vi "RH - PSTC MHCB2 SOFTWARE 2.0.vi"() -> ()   [LabVIEW 2021]
uses:
  Controls/Queue steps Main applic.ctl
  Controls/ApplicSettings.ctl
  <vilib>/Utility/miscctls.llb/LVRectTypeDef.ctl
  Error notification/Controls/Error notification - Settings.ctl
  Error notification/Controls/Error notification - shown buttons.ctl
  Controls/Initialized boards information.ctl
  MDI handling/Controls/MDI FG registered windows states.ctl
  MDI handling/Controls/MDI Arrange child in parent states.ctl
  MDI handling/MDI global.vi
  Controls/RH PSTC MHCB2 CONSOLE global.vi
  <vilib>/Utility/miscctls.llb/LVPointTypeDef.ctl
panel:
  out "Session loaded":path
  in  "Do not use":bool
  out "close":bool
  out "Opened child ref.":refnum<vi>
  out "Session to load":path
  in  "Debugging info":bool
  out "Child to open":path
  in  "Settings":T1
  in  "Queue steps":T3=enum."idle"
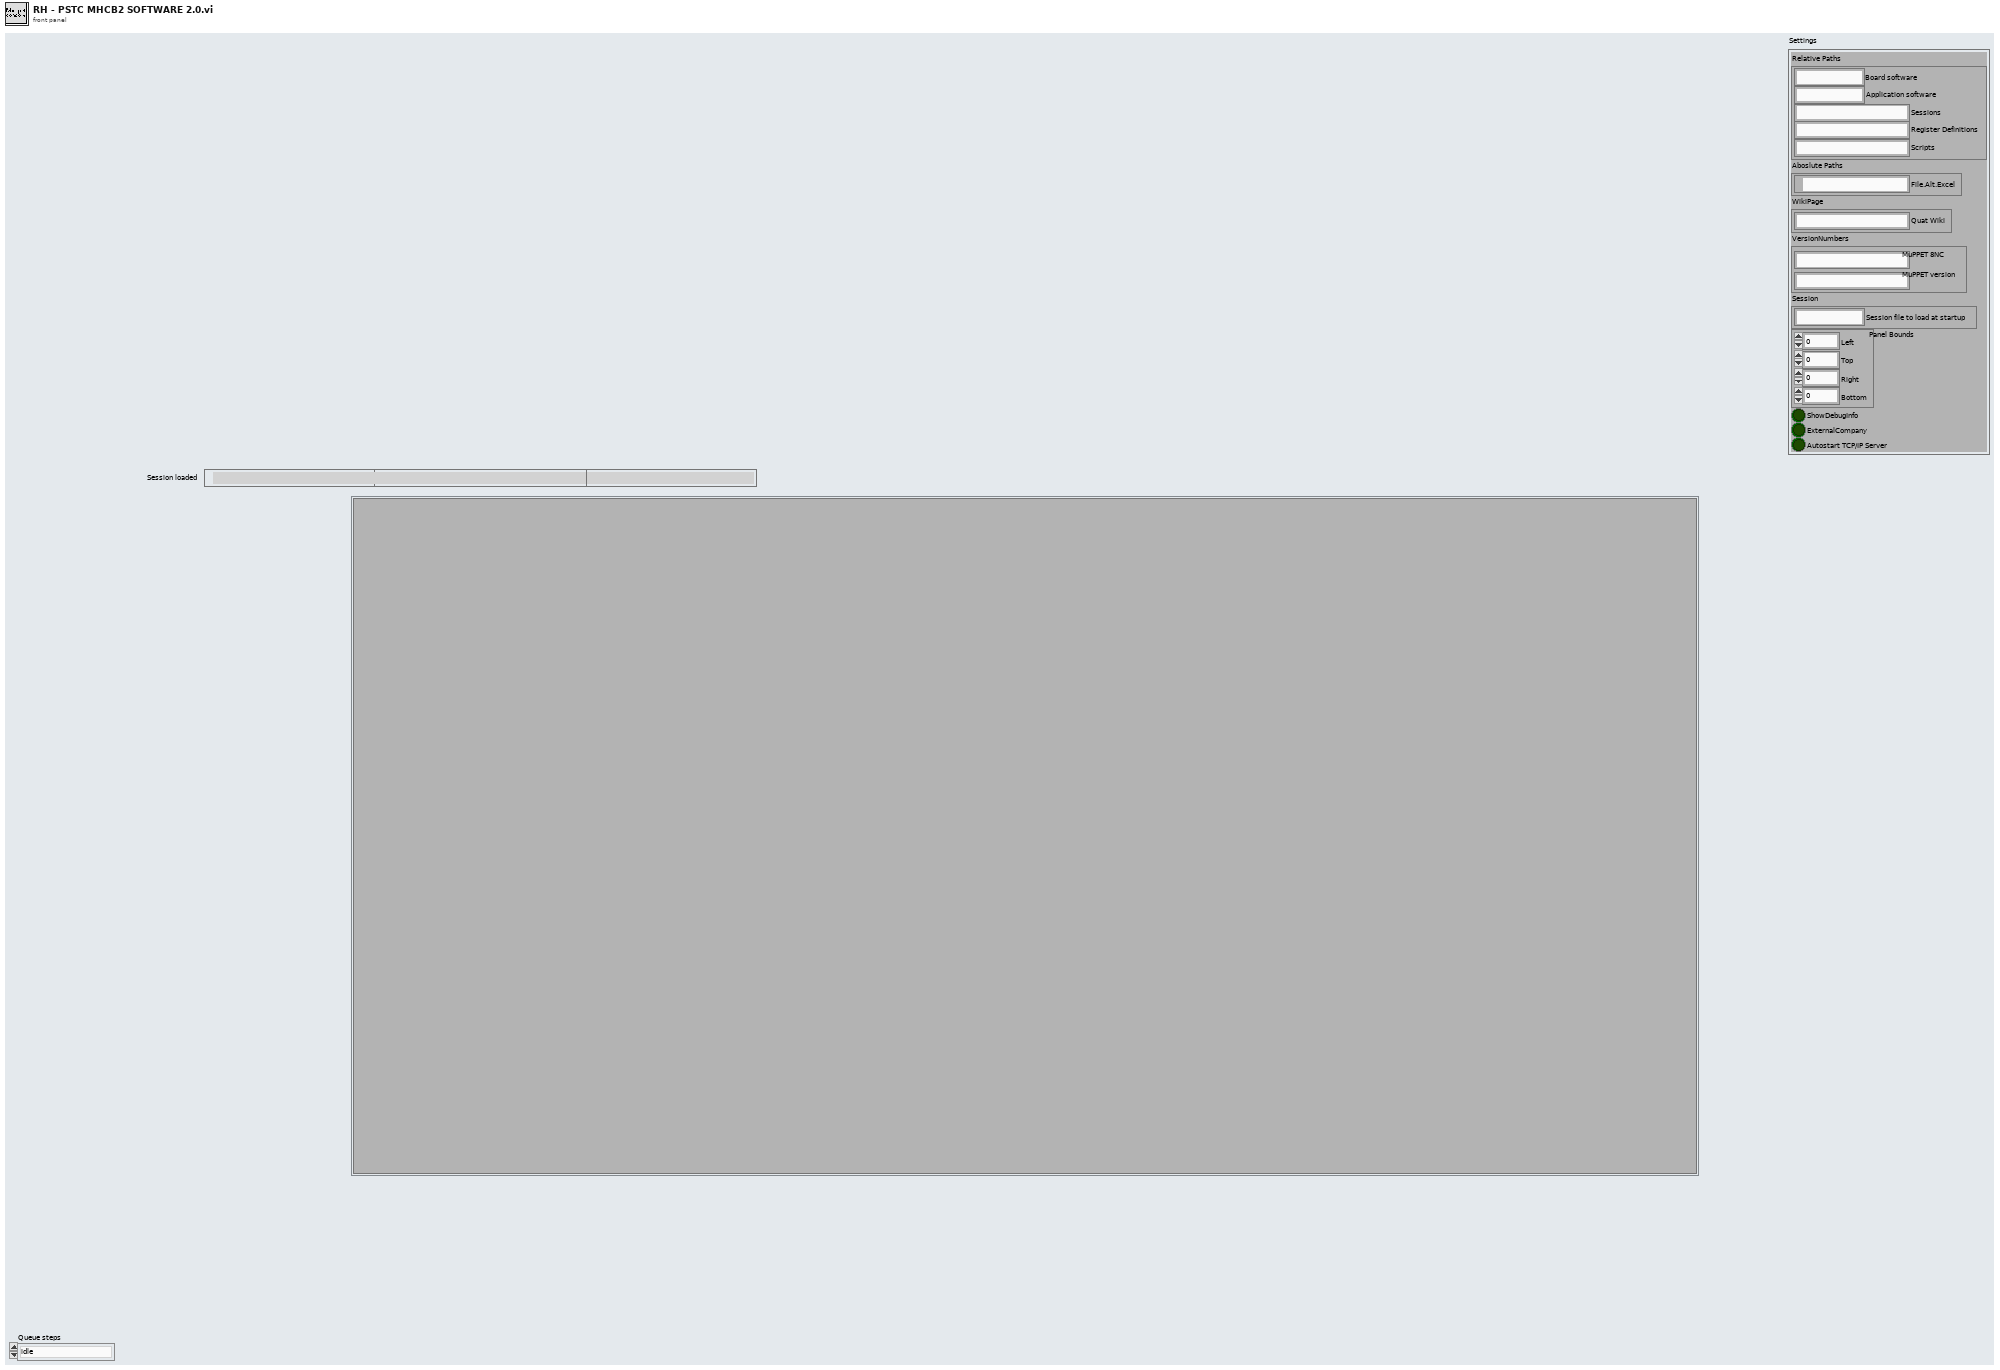
[diagram p1: front panel]
types:
  T1 = typedef "ApplicSettings.ctl" = cluster{"Relative Paths":cluster{"Board software":string, "Application software":string, "Sessions":string, "Register Definitions":string, "Scripts":string}, "Aboslute Paths":cluster{"File.Alt.Excel":path}, "WikiPage":cluster{"Quat Wiki":string}, "VersionNumbers":cluster{"MuPPET 8NC":string, "MuPPET version":string}, "Session":cluster{"Session file to load at startup":string}, "Panel Bounds":T2, "ShowDebugInfo":bool, "ExternalCompany":bool, "Autostart TCP/IP Server":bool}
  T2 = typedef "LVRectTypeDef.ctl" = cluster{"Left":i16, "Top":i16, "Right":i16, "Bottom":i16}
  T3 = typedef "Queue steps Main applic.ctl" = enum16{"init", "idle", "error", "exit", "About", "-----------------", "Startup: Find available software", "Startup: Create pulldown menu", "Startup: Run board SW startup VIs", "File IO: Load applic settings", "File IO: Save applic settings", "MDI: init", "MDI: open child", "MDI: close", "Session: close", "Session: load", "Session: save", "Session: save as", "Hardware: Close", "Script", "TCP IP script server", "Import Excel table layout", "Test: insert error"}
  T4 = enum32{"invalid app kind", "Development System", "Run Time System", "Student Edition", "Embedded LabVIEW", "Evaluation", "Custom"}
  T5 = typedef "Error notification - Settings.ctl" = cluster{"Window Lay-out":cluster{"Title":string, "Show modal":bool, "Default buttons":T6}, "Logging":cluster{"Enable":bool, "Filepath":path, "Max # of lines in file":i32}, "Error definition file":cluster{"Filepath":path}}
  T6 = typedef "Error notification - shown buttons.ctl" = cluster{"Ignore":bool, "Retry":bool, "Abort":bool, "Abort application":bool}
  T7 = typedef "LVPointTypeDef.ctl" = cluster{"Horizontal":i16, "Vertical":i16}
  T8 = typedef "Initialized boards information.ctl" = cluster{"BoardName":string, "Simulation":bool}
  T9 = typedef "MDI FG registered windows states.ctl" = enum16{"init", "add", "replace", "remove", "read"}
  T10 = typedef "MDI Arrange child in parent states.ctl" = enum16{"SW: TopLeft", "SW: Position Coordinated", "SW: Position Incremental", "SW: Center", "SW: Resize", "SW: Resize animated", "AW: Tile", "MW: Arrange Iconic"}
  T11 = cluster{"PositionChildOptions":T10, "X offset":i32, "Y offset":i32}
  T12 = typedef "Error notification - respone.ctl" = enum16{"NOP", "Ignore", "Retry", "Abort", "Abort Applic"}
  T13 = cluster{"IndentLvl":i32, "Type":enum16{"Submenu", "Item", "Separator"}, "Name":string, "Tag":path}[]
  T14 = typedef "MDI child window props.ctl" = cluster{"Owner hWnd":u32, "hWnd":u32, "VI Refnum":refnum<vi>, "WindowTitle":string, "File":string, "Target":string, "RelativeVIPath":string, "PaneState":enum16{"Norm", "Minimized", "Maximized"}}
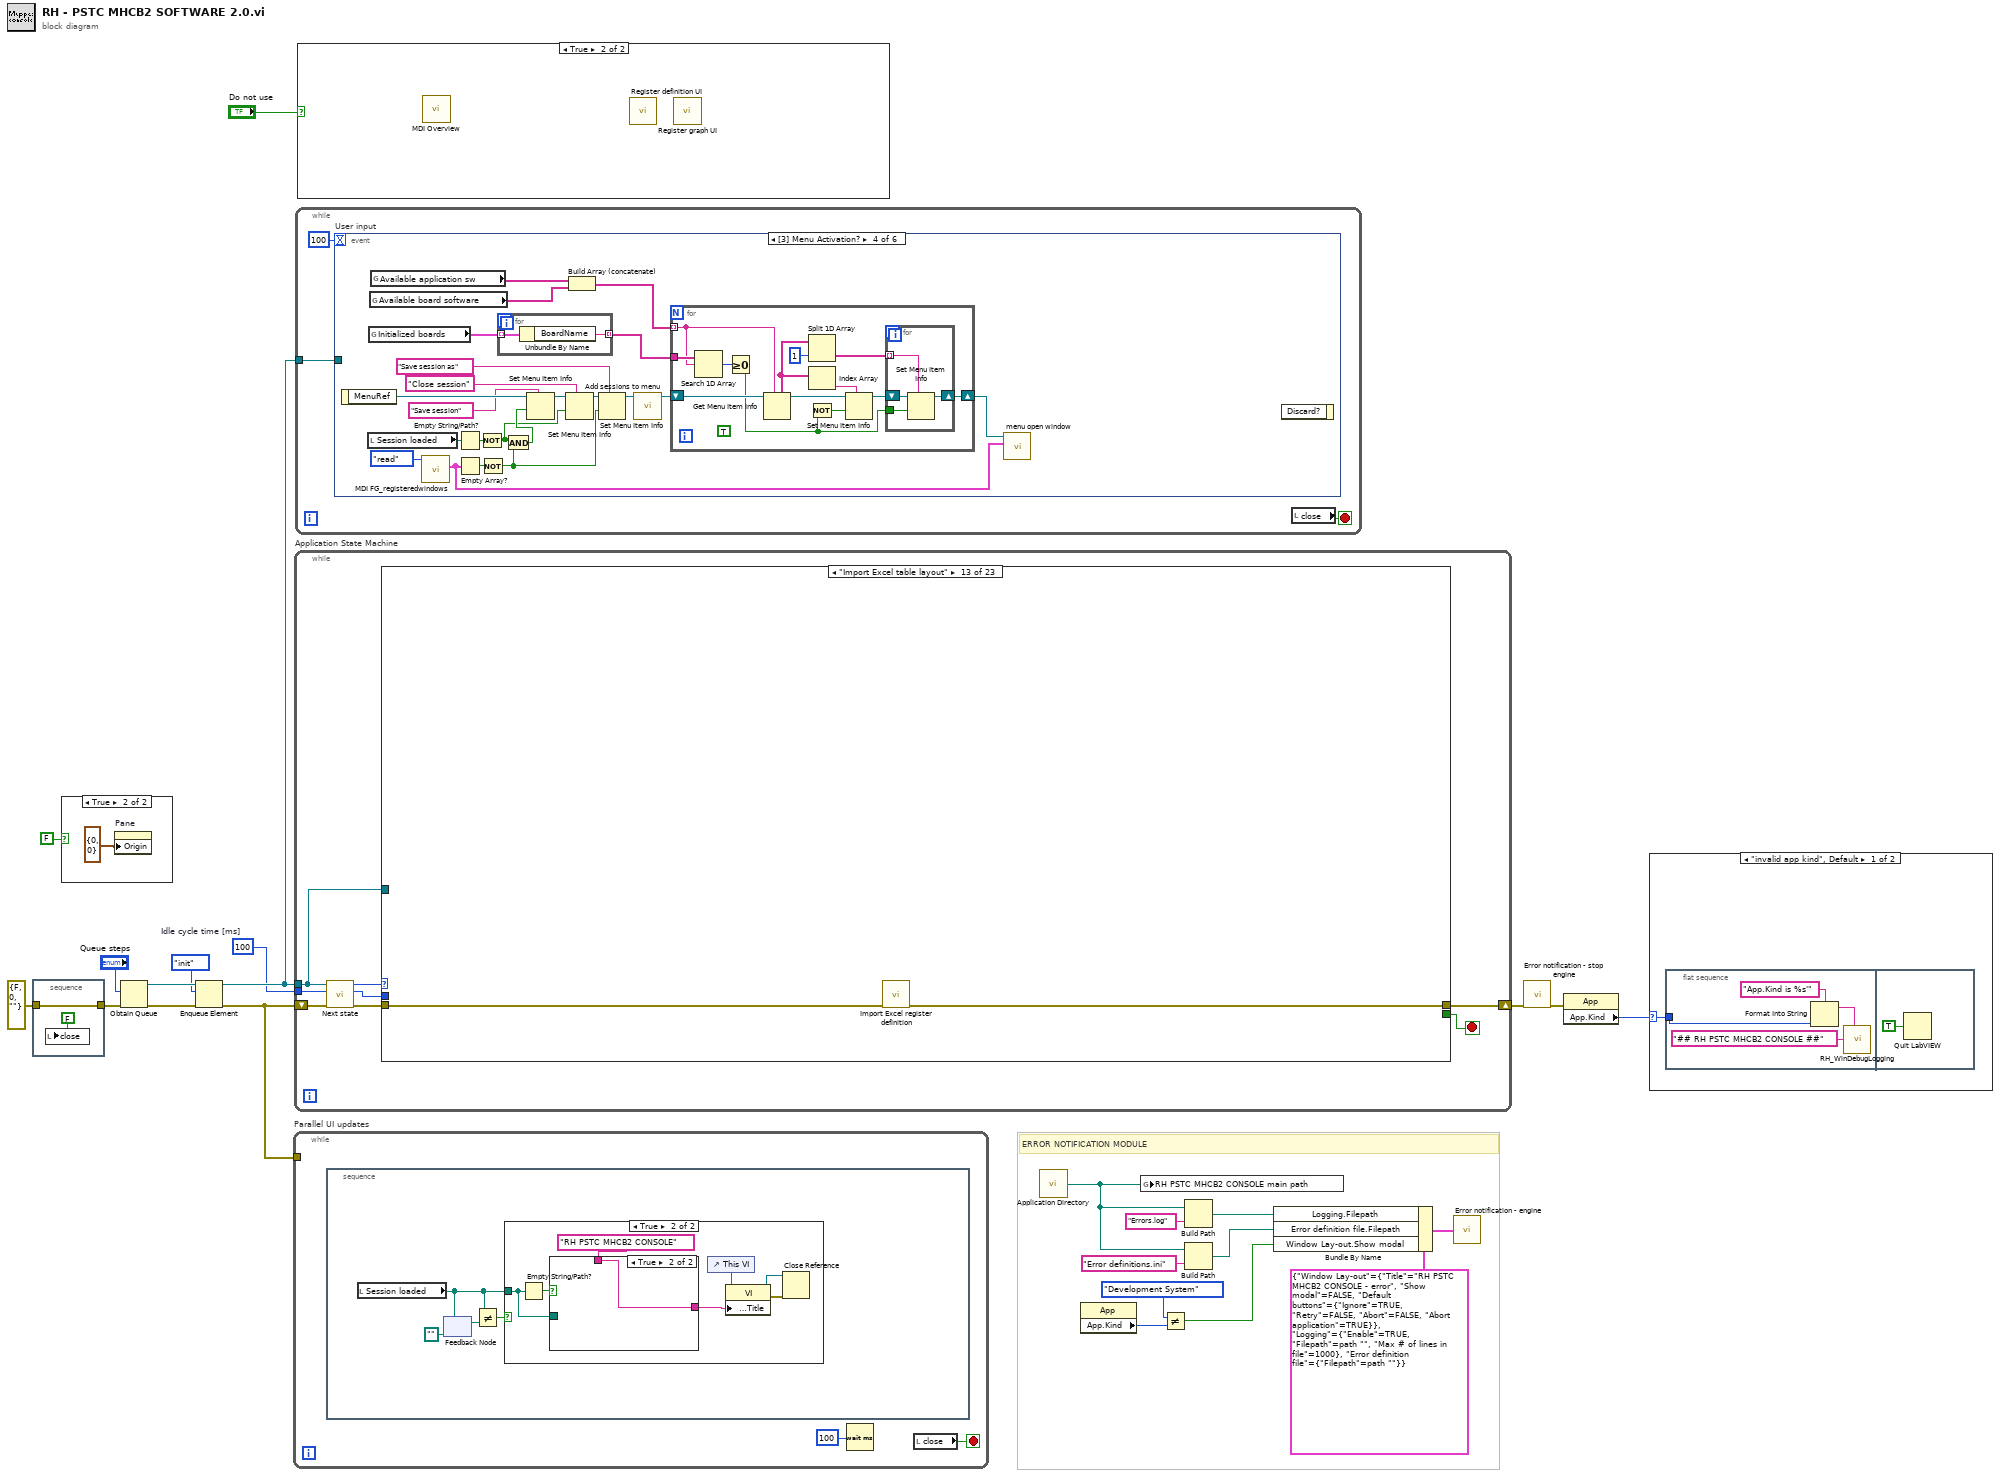
[diagram p0: block diagram]
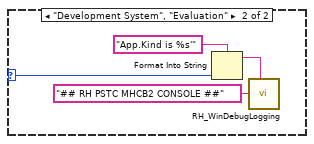
[diagram p3: hidden frame]
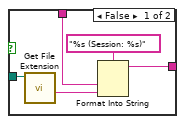
[diagram p5: hidden frame]
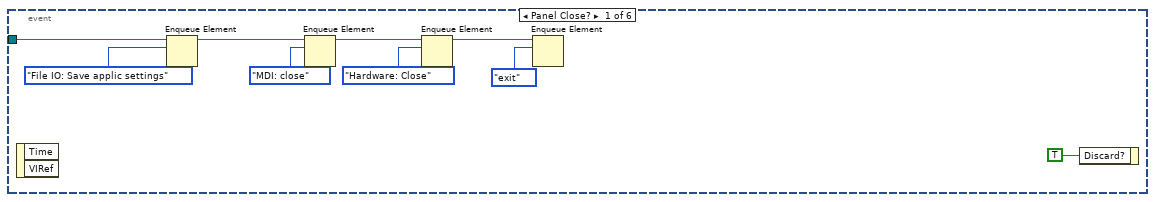
[diagram p7: hidden frame]
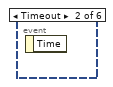
[diagram p8: hidden frame]
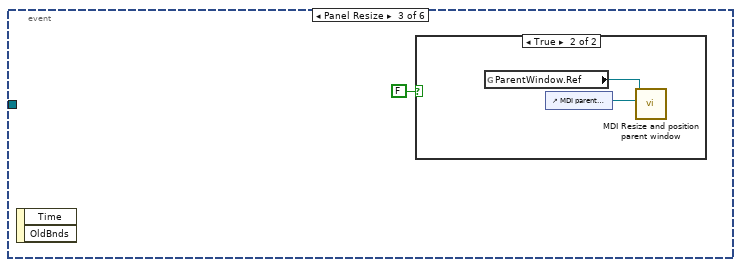
[diagram p9: hidden frame]
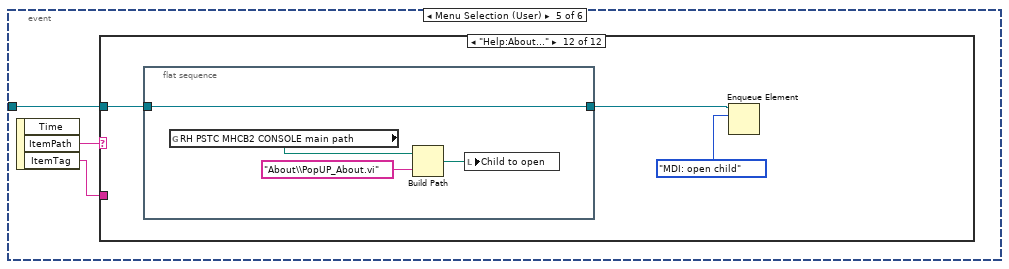
[diagram p11: hidden frame]
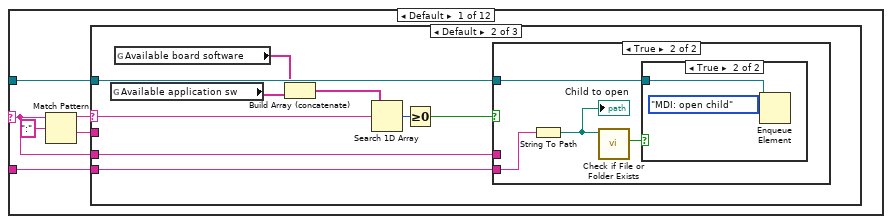
[diagram p12: hidden frame]
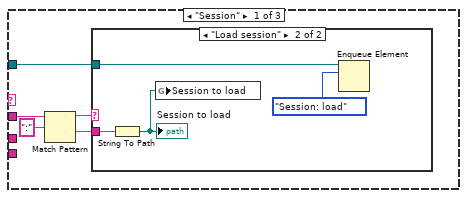
[diagram p13: hidden frame]
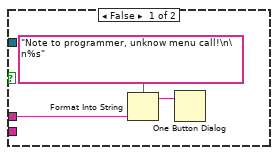
[diagram p15: hidden frame]
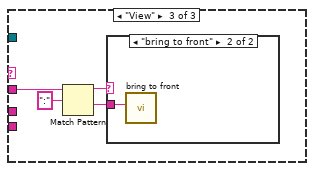
[diagram p17: hidden frame]
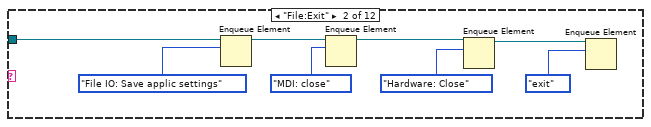
[diagram p19: hidden frame]
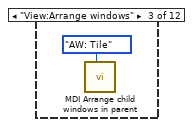
[diagram p20: hidden frame]
diagram:
  w19 = 100  # Idle cycle time [ms]
  # "ERROR NOTIFICATION MODULE"
  n1 = stacked-sequence {
    tunnel: errorcluster {"status"=FALSE, "code"=0, "source"=""} ("error in (no error)") -> [w25]
    tunnel: [w25] -> w16
    frame #0 {
      n2 = local write "close"(FALSE ("close")) -> ()
    }
  }
  n3 = case shown="True" FALSE {
    frame False {
    }
    frame True {
      n4 = property on="Pane" class="Pane"("Origin"=T7 {"Horizontal"=0, "Vertical"=0}) -> ()  [unwired: 2 in, 2 out]
    }
  }
  n5 = Obtain Queue(element data type="Queue steps", error in (no error)=w16) -> (queue out=w23:refnum<queue>, error out=w24:errorcluster)  [unwired: 3 in, 1 out]
  n6 = Enqueue Element(queue=w23, element=Queue_steps_Main_applic."init" ("Queue steps"), error in (no error)=w24) -> (queue out=w20:refnum<queue>, error out=w5:errorcluster)  [unwired: 1 in, 1 out]
  n7 = while "Parallel UI updates" {
    tunnel: w5 -> [_]
    stop <- w28 stop-if-true
    n8 = stacked-sequence {
      frame #0 {
        n9 = local read "Session loaded"() -> (w30:path)
        n10 = feedback #1(path "") -> (w31:path)
        n11 = feedback-in #1(w30) -> ()
        n12 = Not Equal?(x=w30, y=w31) -> (x != y?=w33:bool)
        n13 = case shown="True" w33 {
          tunnel: w30 -> [_ w37]
          frame False {
          }
          frame True {
            n14 = Empty String/Path?(string/path=w37) -> (empty?=w38:bool)
            n15 = case shown="True" w38 {
              tunnel: [w44 w46] -> w39
              tunnel: w37 -> [w43 _]
              tunnel: "RH PSTC MHCB2 CONSOLE" -> [w41 w46]
              frame False {
                n16 = call <vilib>:"Get File Extension.vi"("file"=w43) -> ("filename without extension"=w42:string)  [unwired: 6 in, 4 out]
                n17 = Format Into String(format string="%s (Session: %s)", w41, w42) -> (resulting string=w44:string)  [unwired: 2 in, 1 out]
              }
              frame True {
              }
            }
            n18 = control-ref of="This VI"() -> (w40:refnum<vi>)
            n19 = property class="VI"(reference=w40, "Front Panel.Title"=w39) -> (reference out=w35:refnum<vi>, error out=w36:errorcluster)  [unwired: 1 in]
            n20 = Close Reference(reference=w35, error in (no error)=w36) -> ()  [unwired: 1 out]
          }
        }
      }
    }
    n21 = Wait (ms)(milliseconds to wait=u32 100) -> ()  [unwired: 1 out]
    n22 = local read "close"() -> (w28:bool)
  }
  n23 = while "Application State Machine" {
    shift-right: [w54] -> w3
    shift-left: w5 -> [w48]
    tunnel: w20 -> [w53]
    tunnel: w19 -> [w51]
    stop <- w50 stop-if-true
    n24 = call "Next state.vi"("error in (no error)"=w48, "Idle cycle time [ms]"=w51, "Queue in"=w53) -> ("error out"=w52:errorcluster, "Previous state"=w47:T3, "Next state"=w49:T3)  [unwired: 6 in]
    n25 = case shown="\"Import Excel table layout\"" w49 {
      tunnel: w52 -> [w62 w72 w75 w95 w100 w101 w114 w141 w174 w221 w250 w260 w328 w346 w361 w364 w382 w389 w430 w441 w475 w476 w477]
      tunnel: [w62 w72 w73 w94 w100 w101 w102 w140 w165 w218 w251 w259 w327 w345 w360 w364 w380 w397 w429 w440 w474 w476 w477] -> w54
      tunnel: w53 -> [w65 _ w78 w96 _ _ _ _ _ w216 _ _ _ _ _ _ _ _ _ _ _ _ _]
      tunnel: [_ _ _ w99 _ _ _ _ _ _ _ _ _ _ _ _ _ _ _ _ _ _ _] -> w50
      tunnel: w47 -> [_ _ w74 _ _ _ _ _ _ _ _ _ _ _ _ _ _ _ _ _ _ _ _]
      frame "init" {
        w58 = path "" ("Session to load")
        w64 = T3[] [enum."File IO: Load applic settings", enum."Startup: Find available software", enum."Startup: Create pulldown menu", enum."MDI: init", enum."Startup: Run board SW startup VIs"] items=["init", "idle", "error", "exit", "About", "-----------------", "Startup: Find available software", "Startup: Create pulldown menu", "Startup: Run board SW startup VIs", "File IO: Load applic settings", "File IO: Save applic settings", "MDI: init", "MDI: open child", "MDI: close", "Session: close", "Session: load", "Session: save", "Session: save as", "Hardware: Close", "Script", "TCP IP script server", "Import Excel table layout", "Test: insert error"]
        n26 = case shown="True" FALSE {
          frame False {
          }
          frame True {
            n27 = control-ref of="MDI parent bounds"() -> (w66:refnum<vi>)
            n28 = invoke class="SubPnl" method="FitControlToPane"(reference=w66) -> ()  [unwired: 2 in, 3 out]
          }
        }
        n29 = for {
          tunnel: w65 -> [w71]
          tunnel: w64 -> [w70] mode=indexing
          n30 = Enqueue Element(queue=w71, element=w70) -> ()  [unwired: 2 in, 3 out]
        }
        n31 = call <vilib>:"Application Directory.vi"() -> ("Application Directory"=w60:path)
        n32 = global write "RH PSTC MHCB2 CONSOLE global.vi" "RH PSTC MHCB2 CONSOLE main path"(w60) -> ()
        n33 = local write "Session loaded"(w58) -> ()
        n34 = local write "Session to load"(w58) -> ()
        n35 = property on="MDI parent bounds" class="SubPnl"("Visible"=FALSE) -> ()  [unwired: 2 in, 2 out]
        n36 = case shown="True" FALSE {
          frame False {
          }
          frame True {
            n37 = global read "MDI global.vi" "ParentWindow.Ref"() -> (w69:refnum<vi>)
            n38 = invoke class="VI" method="FP.Close"(reference=w69) -> (error out=w68:errorcluster)  [unwired: 2 in, 2 out]
            n39 = invoke class="VI" method="Abort VI"(reference=w69, error in=w68) -> (error out=w67:errorcluster)  [unwired: 1 in, 2 out]
            n40 = stacked-sequence {
              tunnel: w67 -> [_]
              frame #0 {
              }
            }
          }
        }
        n41 = global write "RH PSTC MHCB2 CONSOLE global.vi" "Initialized boards"(T8[] [] ("Initialized boards")) -> ()
        n42 = global write "RH PSTC MHCB2 CONSOLE global.vi" "Debug - Filepath of files to open"(path[] [] ("Filepath of files to open")) -> ()
        n43 = global write "RH PSTC MHCB2 CONSOLE global.vi" "Session to load"(path "" ("Session to load")) -> ()
      }
      frame "idle" {
      }
      frame "error" {
        n44 = call "Error notification - insert error.vi"("error in (no error)"=w75, "Overrule default shown buttons"=T6 {"Ignore"=TRUE, "Retry"=TRUE, "Abort"=FALSE, "Abort application"=TRUE}, "Current state of state machine (Enum)"=w74) -> ("Response"=w76:T12)  [unwired: 8 in]
        n45 = case shown="\"Abort\", \"Abort Applic\"" w76 {
          tunnel: w78 -> [_ _ w83 w86]
          tunnel: w75 -> [_ _ _ _]
          tunnel: w74 -> [_ _ w82 _]
          tunnel: [w79 w80 w81 w84] -> w73
          frame "NOP" {
            # "Not used"
            n46 = call <vilib>:"Clear Errors.vi"() -> ("error out"=w79:errorcluster)  [unwired: 6 in, 1 out]
          }
          frame "Ignore" {
            n47 = call <vilib>:"Clear Errors.vi"() -> ("error out"=w80:errorcluster)  [unwired: 6 in, 1 out]
          }
          frame "Retry" {
            # "Retry case that caused the error.\nInsert the element in front of the queue."
            n48 = Enqueue Element At Opposite End(queue=w83, element=w82) -> ()  [unwired: 2 in, 3 out]
            n49 = call <vilib>:"Clear Errors.vi"() -> ("error out"=w81:errorcluster)  [unwired: 6 in, 1 out]
          }
          frame "Abort", "Abort Applic" {
            n50 = Flush Queue(queue=w86) -> (queue out=w85:refnum<queue>)  [unwired: 1 in, 2 out]
            n51 = Enqueue Element(queue=w85, element=Queue_steps_Main_applic."File IO: Save applic settings" ("Queue steps")) -> (queue out=w87:refnum<queue>)  [unwired: 2 in, 2 out]
            n52 = Enqueue Element(queue=w87, element=Queue_steps_Main_applic."MDI: close" ("Queue steps")) -> (queue out=w91:refnum<queue>)  [unwired: 2 in, 2 out]
            n53 = call <vilib>:"Clear Errors.vi"() -> ("error out"=w84:errorcluster)  [unwired: 6 in, 1 out]
            n54 = Enqueue Element(queue=w91, element=Queue_steps_Main_applic."Hardware: Close" ("Queue steps")) -> (queue out=w90:refnum<queue>)  [unwired: 2 in, 2 out]
            n55 = Enqueue Element(queue=w90, element=Queue_steps_Main_applic."exit" ("Queue steps")) -> ()  [unwired: 2 in, 3 out]
          }
        }
      }
      frame "exit" {
        w99 = TRUE
        n56 = Release Queue(queue=w96, force destroy? (F)=TRUE, error in (no error)=w95) -> (error out=w94:errorcluster)  [unwired: 2 out]
        n57 = property on="MDI parent bounds" class="SubPnl"("Visible"=TRUE) -> ()  [unwired: 2 in, 2 out]
        "close" <- w99
      }
      frame "About" {
      }
      frame "-----------------" {
      }
      frame "Startup: Find available software" {
        n58 = global read "RH PSTC MHCB2 CONSOLE global.vi" "ApplicSettings"() -> (w118:T1)
        n59 = Unbundle By Name(w118) -> ("Relative Paths.Board software"=w117:string, "Relative Paths.Application software"=w116:string)
        n60 = global read "RH PSTC MHCB2 CONSOLE global.vi" "RH PSTC MHCB2 CONSOLE main path"() -> (w115:path)
        n61 = Build Path(base path=w115, name or relative path=w117) -> (appended path=w104:path)
        n62 = Build Path(base path=w115, name or relative path=w116) -> (appended path=w113:path)
        n63 = call <vilib>:"Check if File or Folder Exists.vi"("error in (no error)"=w114, "path"=w113) -> ("error out"=w111:errorcluster, "file or folder exists?"=w110:bool, "dup path"=w112:path)  [unwired: 7 in]
        n64 = case shown="True" w110 {
          tunnel: w112 -> [_ w130]
          tunnel: w111 -> [w126 w129]
          tunnel: [string[] [] ("folder names") w128] -> w109
          tunnel: [w126 w127] -> w105
          frame False {
          }
          frame True {
            n65 = List Folder(path=w130, error in=w129) -> (folder names=w128:string[], error out=w127:errorcluster)  [unwired: 2 in, 2 out]
          }
        }
        n66 = call <vilib>:"Check if File or Folder Exists.vi"("error in (no error)"=w105, "path"=w104) -> ("error out"=w107:errorcluster, "file or folder exists?"=w108:bool, "dup path"=w106:path)  [unwired: 7 in]
        n67 = case shown="True" w108 {
          tunnel: w106 -> [_ w124]
          tunnel: w107 -> [w120 w123]
          tunnel: [string[] [] ("folder names") w122] -> w103
          tunnel: [w120 w121] -> w102
          frame False {
          }
          frame True {
            n68 = List Folder(path=w124, error in=w123) -> (folder names=w122:string[], error out=w121:errorcluster)  [unwired: 2 in, 2 out]
          }
        }
        n69 = global write "RH PSTC MHCB2 CONSOLE global.vi" "Available application sw"(w109) -> ()
        n70 = global write "RH PSTC MHCB2 CONSOLE global.vi" "Available board software"(w103) -> ()
      }
      frame "Startup: Create pulldown menu" {
        # "PCFMTT"
        # "MINT"
        n71 = global read "RH PSTC MHCB2 CONSOLE global.vi" "ApplicSettings"() -> (w143:T1)
        n72 = Unbundle By Name(w143) -> ("Relative Paths.Board software"=w138:string, "Relative Paths.Application software"=w136:string)
        n73 = global read "RH PSTC MHCB2 CONSOLE global.vi" "Available board software"() -> (w133:string[])
        n74 = global read "RH PSTC MHCB2 CONSOLE global.vi" "Available application sw"() -> (w132:string[])
        n75 = global read "RH PSTC MHCB2 CONSOLE global.vi" "RH PSTC MHCB2 CONSOLE main path"() -> (w139:path)
        n76 = Build Array(w133, w132) -> (w131:string[][])
        n77 = Build Path(base path=w139, name or relative path=w138) -> (appended path=w135:path)
        n78 = Build Path(base path=w139, name or relative path=w136) -> (appended path=w137:path)
        n79 = Build Array(w135, w137) -> (w134:path[])
        n80 = for {
          tunnel: "menu.txt" ("append to path (empty)") -> [w148]
          tunnel: w131 -> [w147] mode=indexing
          tunnel: w134 -> [w144] mode=indexing
          shift-right: [w145] -> w140
          shift-left: w141 -> [w146]
          n81 = for {
            tunnel: w147 -> [w149] mode=indexing
            tunnel: w148 -> [w154]
            shift-right: [w152] -> w145
            shift-left: w146 -> [w153]
            tunnel: w144 -> [w151]
            n82 = Empty String/Path?(string/path=w149) -> (empty?=w150:bool)
            n83 = case shown="False" w150 {
              tunnel: w149 -> [w163 _]
              tunnel: w154 -> [w161 _]
              tunnel: w153 -> [w159 w164]
              tunnel: [w158 w164] -> w152
              tunnel: w151 -> [w155 _]
              frame False {
                n84 = Build Path(base path=w155, name or relative path=w163) -> (appended path=w162:path)
                n85 = Build Path(base path=w162, name or relative path=w161) -> (appended path=w160:path)
                n86 = call "Load menu file.vi"("error in (no error)"=w159, "Menu file path"=w160) -> ("error out"=w158:errorcluster, "MenuItems"=w156:T13)  [unwired: 8 in]
                n87 = Current VI's Menubar() -> (w157:refnum<k9>)
                n88 = call "Add menu items to pulldown menu.vi"("Menu items"=w156, "menu reference"=w157) -> ()  [unwired: 9 in, 1 out]
              }
              frame True {
              }
            }
          }
        }
      }
      frame "Startup: Run board SW startup VIs" {
        n89 = global read "RH PSTC MHCB2 CONSOLE global.vi" "ApplicSettings"() -> (w176:T1)
        n90 = global read "RH PSTC MHCB2 CONSOLE global.vi" "Available board software"() -> (w167:string[])
        n91 = global read "RH PSTC MHCB2 CONSOLE global.vi" "Available application sw"() -> (w168:string[])
        n92 = Unbundle By Name(w176) -> ("Relative Paths.Board software"=w175:string, "Relative Paths.Application software"=w172:string)
        n93 = global read "RH PSTC MHCB2 CONSOLE global.vi" "RH PSTC MHCB2 CONSOLE main path"() -> (w173:path)
        n94 = Build Array(w167, w168) -> (w166:string[][])
        n95 = Build Path(base path=w173, name or relative path=w175) -> (appended path=w171:path)
        n96 = Build Path(base path=w173, name or relative path=w172) -> (appended path=w170:path)
        n97 = Build Array(w171, w170) -> (w169:path[])
        n98 = for "For all software types" {
          tunnel: w169 -> [w179] mode=indexing
          tunnel: w166 -> [w178] mode=indexing
          shift-right: [w177] -> w165
          shift-left: w174 -> [w180]
          n99 = for "Open each registered software packege folder" {
            tunnel: w179 -> [w185]
            tunnel: w178 -> [w181] mode=indexing
            shift-right: [w183] -> w177
            shift-left: w180 -> [w184]
            n100 = Empty String/Path?(string/path=w181) -> (empty?=w182:bool)
            n101 = case "When not empty element, search for startup vi's" shown="False" w182 {
              tunnel: w185 -> [w193 _]
              tunnel: w181 -> [w192 _]
              tunnel: w184 -> [w189 w212]
              tunnel: [w188 w212] -> w183
              frame False {
                n102 = Build Path(base path=w193, name or relative path=w192) -> (appended path=w191:path)
                n103 = Build Path(base path=w191, name or relative path="Startup") -> (appended path=w187:path)
                n104 = call <vilib>:"Check if File or Folder Exists.vi"("path"=w187) -> ("file or folder exists?"=w186:bool)  [unwired: 8 in, 2 out]
                n105 = case "Run startup VI's" shown="True" w186 {
                  tunnel: w189 -> [w194 w201]
                  tunnel: [w194 w198] -> w188
                  tunnel: w187 -> [_ w195]
                  frame False {
                  }
                  frame True {
                    n106 = List Folder(path=w195, pattern="*.vi", error in=w201) -> (filenames=w197:string[], error out=w199:errorcluster)  [unwired: 1 in, 2 out]
                    n107 = Sort 1D Array(array=w197) -> (sorted array=w196:string[])
                    n108 = for {
                      tunnel: w196 -> [w208] mode=indexing
                      tunnel: w195 -> [w209]
                      shift-right: [w203] -> w198
                      shift-left: w199 -> [w211]
                      n109 = Build Path(base path=w209, name or relative path=w208) -> (appended path=w210:path)
                      n110 = Open VI Reference(vi path=w210, options=16, error in (no error)=w211) -> (vi reference=w207:refnum<vi>, error out=w206:errorcluster)  [unwired: 3 in]
                      n111 = invoke class="VI" method="Run VI"(reference=w207, error in=w206, "Wait until done"=TRUE ("Wait Until Done"), "Auto Dispose Ref"=FALSE ("Auto Dispose Reference")) -> (error out=w203:errorcluster)  [unwired: 1 in, 4 out]
                    }
                  }
                }
              }
              frame True {
              }
            }
          }
        }
      }
      frame "File IO: Load applic settings" {
        n112 = global read "RH PSTC MHCB2 CONSOLE global.vi" "RH PSTC MHCB2 CONSOLE main path"() -> (w215:path)
        n113 = control-ref of="Settings"() -> (w220:refnum<vi>)
        n114 = Build Path(base path=w215, name or relative path="application settings.ini" ("append to path (empty)")) -> (appended path=w213:path)
        n115 = call "Dynamic config file control.vi"("Read/Write (read)"=enum16{"Read data", "Write data"}."Read data", "error in (no error)"=w221, "configuration file path"=w213, "Cluster or Tab control ref."=w220) -> ("error out"=w219:errorcluster)  [unwired: 6 in, 1 out]
        n116 = stacked-sequence {
          tunnel: w219 -> [w229 _ _]
          tunnel: [w229 _ _] -> w218
          tunnel: w216 -> [w223 _ w241]
          frame #0 {
            n117 = Unbundle By Name("Settings") -> ("Relative Paths.Sessions"=w226:string, "Session.Session file to load at startup"=w224:string, "ShowDebugInfo"=w227:bool)
            n118 = global read "RH PSTC MHCB2 CONSOLE global.vi" "RH PSTC MHCB2 CONSOLE main path"() -> (w222:path)
            n119 = global write "MDI global.vi" "ContainerShowsDebugInfo"(w227) -> ()
            n120 = Empty String/Path?(string/path=w224) -> (empty?=w225:bool)
            n121 = global write "RH PSTC MHCB2 CONSOLE global.vi" "ApplicSettings"("Settings") -> ()
            n122 = case shown="True" w225 {
              tunnel: w226 -> [w232 _]
              tunnel: w224 -> [w236 _]
              tunnel: w223 -> [w234 _]
              tunnel: w222 -> [w231 _]
              frame False {
                n123 = Build Path(base path=w231, name or relative path=w232) -> (appended path=w230:path)
                n124 = Build Path(base path=w230, name or relative path=w236) -> (appended path=w235:path)
                n125 = local write "Session to load"(w235) -> ()
                n126 = Enqueue Element(queue=w234, element=Queue_steps_Main_applic."Session: load") -> ()  [unwired: 2 in, 3 out]
              }
              frame True {
              }
            }
          }
          frame #1 {
            n127 = local read "Settings"() -> (w240:T1)
            n128 = Unbundle By Name(w240) -> ("Panel Bounds"=w239:T2)
            n129 = call "Resize FP to minimum.vi"("Panel Bounds in"=w239) -> ("Panel Bounds out"=w238:T2)  [unwired: 10 in]
            n130 = control-ref of="This VI"() -> (w237:refnum<vi>)
            n131 = property class="VI"(reference=w237, "Front Panel.PanelBounds"=w238) -> ()  [unwired: 1 in, 2 out]
          }
          frame #2 {
            n132 = global read "RH PSTC MHCB2 CONSOLE global.vi" "ApplicSettings"() -> (w243:T1)
            n133 = Unbundle By Name(w243) -> ("Autostart TCP/IP Server"=w242:bool)
            n134 = case shown="False" w242 {
              tunnel: w241 -> [_ w244]
              frame False {
              }
              frame True {
                n135 = Enqueue Element(queue=w244, element=Queue_steps_Main_applic."TCP IP script server") -> ()  [unwired: 2 in, 3 out]
              }
            }
          }
        }
      }
      frame "File IO: Save applic settings" {
        n136 = stacked-sequence {
          tunnel: w250 -> [w258]
          tunnel: [w258] -> w249
          frame #0 {
            n137 = control-ref of="This VI"() -> (w257:refnum<vi>)
            n138 = global read "RH PSTC MHCB2 CONSOLE global.vi" "ApplicSettings"() -> (w256:T1)
            n139 = property class="VI"(reference=w257) -> ("Front Panel.PanelBounds"=w254:T2)  [unwired: 1 in, 2 out]
            n140 = Bundle By Name(cluster=w256, "Panel Bounds"=w254) -> (w255:T1)
            n141 = local write "Settings"(w255) -> ()
          }
        }
        n142 = global read "RH PSTC MHCB2 CONSOLE global.vi" "RH PSTC MHCB2 CONSOLE main path"() -> (w248:path)
        n143 = control-ref of="Settings"() -> (w252:refnum<vi>)
        n144 = Build Path(base path=w248, name or relative path="application settings.ini" ("append to path (empty)")) -> (appended path=w246:path)
        n145 = call "Dynamic config file control.vi"("Read/Write (read)"=enum16{"Read data", "Write data"}."Write data", "error in (no error)"=w249, "configuration file path"=w246, "Cluster or Tab control ref."=w252) -> ("error out"=w251:errorcluster)  [unwired: 6 in, 1 out]
      }
      frame "Hardware: Close" {
        n146 = disable-structure shown="Enabled" {
          disable-tunnel: w260 -> [w267 w292]
          disable-tunnel: [w266 w293] -> w259
          frame Disabled {
            n147 = global read "RH PSTC MHCB2 CONSOLE global.vi" "MuPPET main path"() -> (w263)
            n148 = global read "RH PSTC MHCB2 CONSOLE global.vi" "ApplicSettings"() -> (w264:T1)
            n149 = global read "RH PSTC MHCB2 CONSOLE global.vi" "Initialized boards"() -> (w265:T8[])
            n150 = Unbundle By Name(w264) -> ("Relative Paths.Board software"=w262:string)
            n151 = Build Path(base path=w263, name or relative path=w262) -> (appended path=w261:path)
            n152 = for "Initialize used boards" {
              shift-right: [w278] -> w266
              shift-left: w267 -> [w275]
              tunnel: w265 -> [w270] mode=indexing
              tunnel: w261 -> [w277]
              n153 = Unbundle By Name(w270) -> ("BoardName"=w269:string)
              n154 = Concatenate Strings(w269, " Close.vi") -> (w272:string)
              n155 = Build Path(base path=w277, name or relative path=w269) -> (appended path=w276:path)
              n156 = call "Initialized Boards -  de(register).vi"("Name of board"=w269, "Register board"=FALSE ("Add board")) -> ()  [unwired: 10 in]
              n157 = Build Path(base path=w276, name or relative path=w272) -> (appended path=w271:path)
              n158 = call <vilib>:"Check if File or Folder Exists.vi"("path"=w271) -> ("file or folder exists?"=w274:bool)  [unwired: 8 in, 2 out]
              n159 = case "When close VI exists, execute it." shown="True" w274 {
                tunnel: w275 -> [w279 w287]
                tunnel: [w279 w286] -> w278
                tunnel: w271 -> [_ w280]
                frame False {
                }
                frame True {
                  n160 = Open VI Reference(vi path=w280, error in (no error)=w287) -> (vi reference=w281:refnum<vi>, error out=w285:errorcluster)  [unwired: 4 in]
                  n161 = invoke class="VI" method="Run VI"(reference=w281, error in=w285, "Wait until done"=TRUE, "Auto Dispose Ref"=FALSE ("Auto Dispose Reference")) -> (error out=w284:errorcluster)  [unwired: 1 in, 4 out]
                  n162 = Close Reference(reference=w281, error in (no error)=w284) -> (error out=w286:errorcluster)
                }
              }
            }
          }
          frame Enabled {
            n163 = global read "RH PSTC MHCB2 CONSOLE global.vi" "RH PSTC MHCB2 CONSOLE main path"() -> (w291:path)
            n164 = global read "RH PSTC MHCB2 CONSOLE global.vi" "Initialized boards"() -> (w290:T8[])
            n165 = global read "RH PSTC MHCB2 CONSOLE global.vi" "Available application sw"() -> (w288:string[])
            n166 = for {
              tunnel: w290 -> [w295] mode=indexing
              tunnel: [w294] -> w289 mode=indexing
              n167 = Unbundle By Name(w295) -> ("BoardName"=w294:string)
            }
            n168 = for "Un-Initialize used boards" {
              shift-right: [w317] -> w293
              shift-left: w292 -> [w315]
              tunnel: w291 -> [w305]
              tunnel: w288 -> [w301]
              tunnel: w289 -> [w300] mode=indexing
              n169 = Search 1D Array(1D array=w301, element=w300) -> (index of element=w307:i32)  [unwired: 1 in]
              n170 = Less Than 0?(x=w307) -> (x < 0?=w306:bool)
              n171 = Select(t="Board software", s=w306, f="Application software") -> (s? t:f=w310:string)
              n172 = call "Initialized Boards -  de(register).vi"("Name of board"=w300, "Register board"=FALSE ("Add board")) -> ()  [unwired: 10 in]
              n173 = Build Path(base path=w305, name or relative path=w310) -> (appended path=w302:path)
              n174 = Build Path(base path=w302, name or relative path=w300) -> (appended path=w303:path)
              n175 = Concatenate Strings(w300, " Close.vi") -> (w312:string)
              n176 = Build Path(base path=w303, name or relative path="Modules") -> (appended path=w316:path)
              n177 = Build Path(base path=w316, name or relative path=w312) -> (appended path=w297:path)
              n178 = call <vilib>:"Check if File or Folder Exists.vi"("path"=w297) -> ("file or folder exists?"=w314:bool)  [unwired: 8 in, 2 out]
              n179 = case "When close VI exists, execute it." shown="True" w314 {
                tunnel: w315 -> [w318 w326]
                tunnel: [w318 w319] -> w317
                tunnel: w297 -> [_ w321]
                frame False {
                }
                frame True {
                  n180 = Open VI Reference(vi path=w321, error in (no error)=w326) -> (vi reference=w322:refnum<vi>, error out=w325:errorcluster)  [unwired: 4 in]
                  n181 = invoke class="VI" method="Run VI"(reference=w322, error in=w325, "Wait until done"=TRUE, "Auto Dispose Ref"=FALSE ("Auto Dispose Reference")) -> (error out=w320:errorcluster)  [unwired: 1 in, 4 out]
                  n182 = Close Reference(reference=w322, error in (no error)=w320) -> (error out=w319:errorcluster)
                }
              }
              n183 = Format Into String(format string="Call '%s'", w297) -> (resulting string=w296:string)  [unwired: 2 in, 1 out]
              n184 = call "RH_WinDebugLogging.vi"("message"=w296, "prefix"="## MuPPET ##") -> ()  [unwired: 6 in, 1 out]
            }
          }
        }
      }
      frame "Import Excel table layout" {
        n185 = call "Import Excel register definition.vi"("error in (no error)"=w328) -> ("error out"=w327:errorcluster)  [unwired: 10 in]
      }
      frame "MDI: init" {
        n186 = global read "RH PSTC MHCB2 CONSOLE global.vi" "RH PSTC MHCB2 CONSOLE main path"() -> (w334:path)
        n187 = Build Path(base path=w334, name or relative path="MDI handling\\MDI Parent window.vi" ("append to path (empty)")) -> (appended path=w332:path)
        n188 = case shown="True" TRUE {
          tunnel: w346 -> [w347 w351]
          tunnel: [w347 w350] -> w342
          tunnel: w332 -> [_ w349]
          tunnel: [_ w348] -> w331
          frame False {
          }
          frame True {
            n189 = call "MDI abort and run VI.vi"("Error in (no error)"=w351, "appended path"=w349) -> ("error out"=w350:errorcluster, "VI ref."=w348:refnum<vi>)  [unwired: 8 in]
          }
        }
        n190 = call "MDI Get Window title & handle.vi"("Request handle (F)"=TRUE, "error in (no error)"=w342, "VI Ref."=w331) -> ("error out"=w337:errorcluster, "hWnd"=w338:u32)  [unwired: 6 in, 1 out]
        n191 = case shown="True" TRUE {
          tunnel: w331 -> [_ w352]
          frame False {
          }
          frame True {
            n192 = control-ref of="MDI parent bounds"() -> (w353:refnum<vi>)
            n193 = call "MDI Resize and position parent window.vi"("MDI container bounds"=w353, "VI Ref container"=w352) -> ()  [unwired: 10 in]
          }
        }
        n194 = control-ref of="This VI"() -> (w339:refnum<vi>)
        n195 = call "MDI Get Window title & handle.vi"("Request handle (F)"=TRUE, "error in (no error)"=w337, "VI Ref."=w339) -> ("error out"=w341:errorcluster, "hWnd"=w340:u32)  [unwired: 6 in, 1 out]
        n196 = call "MDI Set Parent Window.vi"("error in (no error)"=w341, "new parent"=w340, "child"=w338) -> ("error out"=w343:errorcluster)  [unwired: 8 in]
        n197 = global write "MDI global.vi" "ParentWindow.Ref"(w331) -> ()
        n198 = global write "MDI global.vi" "MainWindow.Handle"(w340) -> ()
        n199 = global write "MDI global.vi" "ParentWindow.Handle"(w338) -> ()
        n200 = call "MDI FG_registeredwindows.vi"("error in (no error)"=w343, "action"=MDI_FG_registered_windows_states."init") -> ("error out"=w345:errorcluster)  [unwired: 8 in, 1 out]
      }
      frame "MDI: open child" {
        n201 = global read "MDI global.vi" "ParentWindow.Handle"() -> (w357:u32)
        n202 = local read "Child to open"() -> (w355:path)
        n203 = call "MDI Open Child.vi"("error IO"=w361, "Owner hWnd"=w357, "Position Child"=T11 {"PositionChildOptions"=enum."SW: Center", "X offset"=0, "Y offset"=0}, "Path"=w355) -> ("error out"=w360:errorcluster, "Opened child ref."=→"Opened child ref.":refnum<vi>)  [unwired: 5 in, 1 out]
        n204 = global read "RH PSTC MHCB2 CONSOLE global.vi" "Debug - Filepath of files to open"() -> (w356:path[])
        n205 = Insert Into Array(array=w356, new element=w355) -> (w354:path[])  [unwired: 1 in]
        n206 = global write "RH PSTC MHCB2 CONSOLE global.vi" "Debug - Filepath of files to open"(w354) -> ()
      }
      frame "MDI: close" {
        n207 = call "MDI FG_registeredwindows.vi"("error in (no error)"=w364, "action"=MDI_FG_registered_windows_states."read") -> ("error out"=w365:errorcluster, "windows"=w363:T14[])  [unwired: 8 in]
        n208 = Reverse 1D Array(array=w363) -> (reversed array=w362:T14[])
        n209 = for {
          tunnel: w362 -> [w374] mode=indexing
          tunnel: w365 -> [w373]
          tunnel: [w375] -> w367
          n210 = call "MDI Close & deregister window.vi"("error in"=w373, "window"=w374) -> ("error out"=w375:errorcluster)  [unwired: 8 in]
        }
        n211 = global read "MDI global.vi" "ParentWindow.Ref"() -> (w366:refnum<vi>)
        n212 = flat-sequence {
          tunnel: w367 -> [_]
          tunnel: w366 -> [w371]
          tunnel: [w369] -> _
          frame #0 {
            n213 = invoke class="VI" method="FP.Close"(reference=w371) -> (error out=w372:errorcluster)  [unwired: 2 in, 2 out]
            n214 = global write "MDI global.vi" "ParentWindow.Ref"(refnum<k0> refnum) -> ()
            n215 = invoke class="VI" method="Abort VI"(reference=w371, error in=w372) -> (error out=w369:errorcluster)  [unwired: 1 in, 2 out]
          }
        }
      }
      frame "Session: close" {
        # "Remove all windows"
        n216 = call "MDI FG_registeredwindows.vi"("error in (no error)"=w382, "action"=MDI_FG_registered_windows_states."read") -> ("error out"=w383:errorcluster, "windows"=w384:T14[])  [unwired: 8 in]
        n217 = Reverse 1D Array(array=w384) -> (reversed array=w376:T14[])
        n218 = for {
          tunnel: w376 -> [w388] mode=indexing
          tunnel: w383 -> [w387]
          tunnel: [w386] -> w381 mode=indexing
          n219 = call "MDI Close & deregister window.vi"("error in"=w387, "window"=w388) -> ("error out"=w386:errorcluster)  [unwired: 8 in]
        }
        n220 = global write "RH PSTC MHCB2 CONSOLE global.vi" "Session to load"(path "" ("Session to load")) -> ()
        n221 = local write "Session loaded"(path "" ("Session to load")) -> ()
        n222 = global write "RH PSTC MHCB2 CONSOLE global.vi" "Debug - Filepath of files to open"(path[] [] ("Filepath of files to open")) -> ()
        n223 = Merge Errors(w381) -> (w380:errorcluster)
      }
      frame "Session: load" {
        n224 = local read "Session loaded"() -> (w391:path)
        n225 = Empty String/Path?(string/path=w391) -> (empty?=w392:bool)
        n226 = case shown="True" w392 {
          tunnel: [w398 w400] -> w393
          tunnel: w391 -> [w399 _]
          frame False {
            n227 = Strip Path(path=w399) -> (stripped path=w398:path)  [unwired: 1 out]
          }
          frame True {
            n228 = global read "RH PSTC MHCB2 CONSOLE global.vi" "ApplicSettings"() -> (w403:T1)
            n229 = global read "RH PSTC MHCB2 CONSOLE global.vi" "RH PSTC MHCB2 CONSOLE main path"() -> (w402:path)
            n230 = Unbundle By Name(w403) -> ("Relative Paths.Sessions"=w401:string)
            n231 = Build Path(base path=w402, name or relative path=w401) -> (appended path=w400:path)
          }
        }
        n232 = local read "Session to load"() -> (w394:path)
        n233 = Empty String/Path?(string/path=w394) -> (empty?=w396:bool)
        n234 = case "Let user browse" shown="True" w396 {
          tunnel: [w418 w421] -> w395
          tunnel: w394 -> [w418 _]
          tunnel: w393 -> [_ w419]
          tunnel: [FALSE ("cancelled") w427] -> w390
          tunnel: [_ w426] -> _
          frame False {
          }
          frame True {
            n235 = feedback #2 "remember path"(w419) -> (w420:path)
            n236 = call "File Dialog"("start path"=w420, "prompt"="Select session to load", "button label"="Load", "pattern (all files)"="*.session", "pattern label"="MuPPET Session files") -> ("selected path"=w421:path, "cancelled"=w427:bool, "error out"=w426:errorcluster)  [unwired: 7 in, 1 out]
            n237 = feedback-in #2(w421) -> ()
          }
        }
        n238 = case "Cancel pressed?" shown="False" w390 {
          tunnel: [w412 w416] -> w397
          tunnel: w389 -> [w406 w416]
          tunnel: w395 -> [w411 _]
          frame False {
            # "Remove all opened windows"
            # "Load session"
            n239 = call "MDI FG_registeredwindows.vi"("error in (no error)"=w406, "action"=MDI_FG_registered_windows_states."read") -> ("error out"=w409:errorcluster, "windows"=w408:T14[])  [unwired: 8 in]
            n240 = Reverse 1D Array(array=w408) -> (reversed array=w404:T14[])
            n241 = for {
              tunnel: w404 -> [w415] mode=indexing
              tunnel: w409 -> [w414]
              tunnel: [w413] -> w410 mode=indexing
              n242 = call "MDI Close & deregister window.vi"("error in"=w414, "window"=w415) -> ("error out"=w413:errorcluster)  [unwired: 8 in]
            }
            n243 = Merge Errors(w410) -> (w405:errorcluster)
            n244 = call "Load session.vi"("error in (no error)"=w405, "Session to load"=w411) -> ("error out"=w412:errorcluster)  [unwired: 9 in]
            "Session loaded" <- w411
          }
          frame True {
            # "skip load, cancelled by user"
          }
        }
      }
      frame "Session: save" {
        n245 = local read "Session loaded"() -> (w428:path)
        n246 = call "Save session.vi"("error in (no error)"=w430, "Session path"=w428) -> ("error out"=w429:errorcluster)  [unwired: 9 in]
      }
      frame "Session: save as" {
        n247 = local read "Session loaded"() -> (w435:path)
        n248 = Empty String/Path?(string/path=w435) -> (empty?=w434:bool)
        n249 = case shown="True" w434 {
          tunnel: [w446 w452] -> w431
          tunnel: [w445 "New.session" ("name")] -> w436
          tunnel: w435 -> [w447 _]
          frame False {
            n250 = Strip Path(path=w447) -> (stripped path=w446:path, name=w445:string)
          }
          frame True {
            n251 = global read "RH PSTC MHCB2 CONSOLE global.vi" "ApplicSettings"() -> (w449:T1)
            n252 = Unbundle By Name(w449) -> ("Relative Paths.Sessions"=w451:string)
            n253 = global read "RH PSTC MHCB2 CONSOLE global.vi" "RH PSTC MHCB2 CONSOLE main path"() -> (w450:path)
            n254 = Build Path(base path=w450, name or relative path=w451) -> (appended path=w452:path)
          }
        }
        n255 = feedback #3 "remember path"(w431) -> (w432:path)
        n256 = call "File Dialog2"("start path"=w432, "prompt"="Enter session filename", "button label"="Save", "default name"=w436, "error in"=w441, "pattern (all files)"="*.session", "pattern label"="MuPPET Session files") -> ("selected path"=w433:path, "cancelled"=w443:bool, "error out"=w444:errorcluster)  [unwired: 5 in, 1 out]
        n257 = feedback-in #3(w433) -> ()
        n258 = case shown="False" w443 {
          tunnel: w444 -> [w455 w461]
          tunnel: w433 -> [w454 _]
          tunnel: [w453 w460] -> w440
          frame False {
            n259 = case shown="No Error" w455 {
              selector: w455 -> [w458 w459]
              tunnel: w454 -> [w456 _]
              tunnel: [w457 w459] -> w453
              frame No Error {
                n260 = local write "Session loaded"(w456) -> ()
                n261 = call "Save session.vi"("error in (no error)"=w458, "Session path"=w456) -> ("error out"=w457:errorcluster)  [unwired: 9 in]
              }
              frame Error {
              }
            }
          }
          frame True {
            n262 = case shown="Error" w461 {
              selector: w461 -> [w462 w464]
              tunnel: [w462 w463] -> w460
              frame No Error {
              }
              frame Error {
                n263 = Unbundle By Name(w464) -> ("code"=w468:i32)
                n264 = Equal?(x=w468, y=43) -> (x = y?=w465:bool)
                n265 = Select(t=errorcluster {"status"=FALSE, "code"=0, "source"=""} ("error IO"), s=w465, f=w464) -> (s? t:f=w463:errorcluster)
              }
            }
          }
        }
      }
      frame "Script" {
        (unwired) TRUE  # Framework VI
        n266 = global read "MDI global.vi" "ParentWindow.Handle"() -> (w469:u32)
        n267 = global read "RH PSTC MHCB2 CONSOLE global.vi" "RH PSTC MHCB2 CONSOLE main path"() -> (w472:path)
        n268 = Build Path(base path=w472, name or relative path="Modules\\Scripting\\Scripting - Main\\Script Engine - Main.vi" ("append to path (empty)")) -> (appended path=w470:path)
        n269 = call "MDI Open Child.vi"("error IO"=w475, "Owner hWnd"=w469, "Position Child"=T11 {"PositionChildOptions"=enum."SW: Center", "X offset"=0, "Y offset"=0}, "Path"=w470) -> ("error out"=w474:errorcluster)  [unwired: 5 in, 2 out]
      }
      frame "TCP IP script server" {
      }
      frame "Test: insert error" {
      }
    }
  }
  n270 = while {
    tunnel: w20 -> [w480]
    stop <- w478 stop-if-true
    n271 = event "User input" shown="[3] Menu Activation?" {
      selector: _ -> [_ _ _ _ _ _]
      dyn-events: _ -> [_ _ _ _ _ _]
      timeout: 100 -> [_ _ _ _ _ _]
      tunnel: w480 -> [w482 _ _ _ w535 _]
      event Panel Close? {
        n272 = event-data() -> ()  [unwired: 1 in, 2 out]
        n273 = Enqueue Element(queue=w482, element=Queue_steps_Main_applic."File IO: Save applic settings" ("Queue steps")) -> (queue out=w481:refnum<queue>)  [unwired: 2 in, 2 out]
        n274 = Enqueue Element(queue=w481, element=Queue_steps_Main_applic."MDI: close" ("Queue steps")) -> (queue out=w486:refnum<queue>)  [unwired: 2 in, 2 out]
        n275 = Enqueue Element(queue=w486, element=Queue_steps_Main_applic."Hardware: Close" ("Queue steps")) -> (queue out=w485:refnum<queue>)  [unwired: 2 in, 2 out]
        n276 = Enqueue Element(queue=w485, element=Queue_steps_Main_applic."exit" ("Queue steps")) -> ()  [unwired: 2 in, 3 out]
        n277 = event-data("Discard?"=TRUE) -> ()  [unwired: 1 in, 1 out]
      }
      event Timeout {
        n278 = event-data() -> ()  [unwired: 1 in, 1 out]
      }
      event Panel Resize {
        n279 = event-data() -> ()  [unwired: 1 in, 2 out]
        n280 = case shown="True" FALSE {
          frame False {
          }
          frame True {
            n281 = global read "MDI global.vi" "ParentWindow.Ref"() -> (w492:refnum<vi>)
            n282 = control-ref of="MDI parent bounds"() -> (w491:refnum<vi>)
            n283 = call "MDI Resize and position parent window.vi"("MDI container bounds"=w491, "VI Ref container"=w492) -> ()  [unwired: 10 in]
          }
        }
      }
      event Menu Activation? {
        n284 = event-data() -> ("MenuRef"=w511:refnum<k9>)  [unwired: 1 in]
        n285 = local read "Session loaded"() -> (w509:path)
        n286 = global read "RH PSTC MHCB2 CONSOLE global.vi" "Initialized boards"() -> (w513:T8[])
        n287 = global read "RH PSTC MHCB2 CONSOLE global.vi" "Available board software"() -> (w496:string[])
        n288 = global read "RH PSTC MHCB2 CONSOLE global.vi" "Available application sw"() -> (w497:string[])
        n289 = call "MDI FG_registeredwindows.vi"("action"=MDI_FG_registered_windows_states."read") -> ("windows"=w494:T14[])  [unwired: 9 in, 1 out]
        n290 = Empty String/Path?(string/path=w509) -> (empty?=w510:bool)
        n291 = Empty Array?(array=w494) -> (empty?=w506:bool)
        n292 = Not(x=w510) -> (.not. x?=w498:bool)
        n293 = Not(x=w506) -> (.not. x?=w500:bool)
        n294 = for {
          tunnel: w513 -> [w516] mode=indexing
          tunnel: [w515] -> w512 mode=indexing
          n295 = Unbundle By Name(w516) -> ("BoardName"=w515:string)
        }
        n296 = And(x=w498, y=w500) -> (x .and. y?=w499:bool)
        n297 = Set Menu Item Info(7:"Save session" ("item name"), 9:w499, 11:w511) -> (3:w507:refnum<k9>)  [unwired: 4 in, 1 out]
        n298 = Set Menu Item Info(7:"Close session" ("item name"), 9:w498, 11:w507) -> (3:w503:refnum<k9>)  [unwired: 4 in, 1 out]
        n299 = Build Array (concatenate)(w497, w496) -> (w495:string[])
        n300 = Set Menu Item Info(7:"Save session as" ("item name"), 9:w500, 11:w503) -> (3:w502:refnum<k9>)  [unwired: 4 in, 1 out]
        n301 = call "Add sessions to menu.vi"("Menu Refnum"=w502) -> ("Menu ref. dup"=w514:refnum<k9>)  [unwired: 10 in]
        n302 = for {
          tunnel: w495 -> [w526] mode=indexing
          tunnel: w512 -> [w529]
          shift-right: [w517] -> w493
          shift-left: w514 -> [w527]
          (unwired) TRUE
          n303 = Search 1D Array(1D array=w529, element=w526) -> (index of element=w528:i32)  [unwired: 1 in]
          n304 = Greater Or Equal To 0?(x=w528) -> (x >= 0?=w518:bool)
          n305 = Get Menu Item Info(7:w526, 11:w527) -> (3:w525:refnum<k9>, 5:w523:string[])  [unwired: 1 in, 5 out]
          n306 = Split 1D Array(array=w523, index=1) -> (second subarray=w521:string[])  [unwired: 1 out]
          n307 = Index Array(array=w523) -> (element=w522:string)  [unwired: 1 in]
          n308 = Not(x=w518) -> (.not. x?=w519:bool)
          n309 = Set Menu Item Info(7:w522, 9:w519, 11:w525) -> (3:w520:refnum<k9>)  [unwired: 4 in, 1 out]
          n310 = for {
            tunnel: w521 -> [w532] mode=indexing
            tunnel: w518 -> [w531]
            shift-right: [w530] -> w517
            shift-left: w520 -> [w533]
            n311 = Set Menu Item Info(7:w532, 9:w531, 11:w533) -> (3:w530:refnum<k9>)  [unwired: 4 in, 1 out]
          }
        }
        n312 = call "menu open window.vi"("windows"=w494, "Menu in"=w493) -> ()  [unwired: 8 in, 2 out]
        n313 = event-data() -> ()  [unwired: 2 in, 1 out]
      }
      event Menu Selection (User) {
        n314 = event-data() -> ("ItemPath"=w536:string, "ItemTag"=w534:string)  [unwired: 1 in, 1 out]
        n315 = case shown="\"Help:About...\"" w536 {
          selector: w536 -> [w538 _ _ _ _ _ _ _ _ _ _ _]
          tunnel: w535 -> [w542 w576 _ _ w592 w594 w596 w598 w603 w605 w607 w609]
          tunnel: w534 -> [w537 _ _ _ _ _ _ _ _ _ _ _]
          frame Default {
            n316 = Match Pattern(string=w538, regular expression=":") -> (before substring=w540:string, after substring=w539:string)  [unwired: 1 in, 2 out]
            n317 = case shown="Default" w540 {
              selector: w540 -> [_ w557 _]
              tunnel: w542 -> [w544 w560 _]
              tunnel: w539 -> [w543 _ w572]
              tunnel: w538 -> [_ w556 _]
              tunnel: w537 -> [_ w555 _]
              frame "Session" {
                n318 = Match Pattern(string=w543, regular expression=":") -> (before substring=w546:string, after substring=w545:string)  [unwired: 1 in, 2 out]
                n319 = case shown="\"Load session\"" w546 {
                  tunnel: w545 -> [_ w551]
                  tunnel: w544 -> [_ w548]
                  frame Default {
                  }
                  frame "Load session" {
                    n320 = String To Path(string=w551) -> (path=w549:path)
                    "Session to load" <- w549
                    n321 = global write "RH PSTC MHCB2 CONSOLE global.vi" "Session to load"(w549) -> ()
                    n322 = Enqueue Element(queue=w548, element=Queue_steps_Main_applic."Session: load") -> ()  [unwired: 2 in, 3 out]
                  }
                }
              }
              frame Default {
                n323 = global read "RH PSTC MHCB2 CONSOLE global.vi" "Available application sw"() -> (w553:string[])
                n324 = global read "RH PSTC MHCB2 CONSOLE global.vi" "Available board software"() -> (w554:string[])
                n325 = Build Array (concatenate)(w554, w553) -> (w552:string[])
                n326 = Search 1D Array(1D array=w552, element=w557) -> (index of element=w559:i32)  [unwired: 1 in]
                n327 = Greater Or Equal To 0?(x=w559) -> (x >= 0?=w558:bool)
                n328 = case shown="True" w558 {
                  tunnel: w560 -> [_ w565]
                  tunnel: w556 -> [w561 _]
                  tunnel: w555 -> [_ w564]
                  frame False {
                    n329 = Format Into String(format string="Note to programmer, unknow menu call!\n\n%s" ("message"), w561) -> (resulting string=w562:string)  [unwired: 2 in, 1 out]
                    n330 = One Button Dialog(message=w562) -> ()  [unwired: 1 in, 1 out]
                  }
                  frame True {
                    n331 = String To Path(string=w564) -> (path=w567:path)
                    "Child to open" <- w567
                    n332 = call <vilib>:"Check if File or Folder Exists.vi"("path"=w567) -> ("file or folder exists?"=w566:bool)  [unwired: 8 in, 2 out]
                    n333 = case shown="True" w566 {
                      tunnel: w565 -> [_ w568]
                      frame False {
                        # "create error here"
                      }
                      frame True {
                        n334 = Enqueue Element(queue=w568, element=Queue_steps_Main_applic."MDI: open child") -> ()  [unwired: 2 in, 3 out]
                      }
                    }
                  }
                }
              }
              frame "View" {
                n335 = Match Pattern(string=w572, regular expression=":") -> (before substring=w571:string, after substring=w570:string)  [unwired: 1 in, 2 out]
                n336 = case shown="\"bring to front\"" w571 {
                  tunnel: w570 -> [_ w574]
                  frame "False", Default {
                    # "#todo\nwindow is undifinde\nalso make this output \nfrom other cases"
                  }
                  frame "bring to front" {
                    n337 = call "bring to front.vi"("to front name"=w574) -> ()  [unwired: 11 in]
                  }
                }
              }
            }
          }
          frame "File:Exit" {
            n338 = Enqueue Element(queue=w576, element=Queue_steps_Main_applic."File IO: Save applic settings" ("Queue steps")) -> (queue out=w575:refnum<queue>)  [unwired: 2 in, 2 out]
            n339 = Enqueue Element(queue=w575, element=Queue_steps_Main_applic."MDI: close" ("Queue steps")) -> (queue out=w579:refnum<queue>)  [unwired: 2 in, 2 out]
            n340 = Enqueue Element(queue=w579, element=Queue_steps_Main_applic."Hardware: Close" ("Queue steps")) -> (queue out=w578:refnum<queue>)  [unwired: 2 in, 2 out]
            n341 = Enqueue Element(queue=w578, element=Queue_steps_Main_applic."exit" ("Queue steps")) -> ()  [unwired: 2 in, 3 out]
          }
          frame "View:Arrange windows" {
            n342 = call "MDI Arrange child windows in parent.vi"("PositionChildOptions"=MDI_Arrange_child_in_parent_states."AW: Tile") -> ()  [unwired: 10 in, 1 out]
          }
          frame "View:Close all windows" {
            n343 = call "MDI FG_registeredwindows.vi"("action"=MDI_FG_registered_windows_states."read") -> ("error out"=w587:errorcluster, "windows"=w585:T14[])  [unwired: 9 in]
            n344 = Reverse 1D Array(array=w585) -> (reversed array=w584:T14[])
            n345 = for {
              tunnel: w584 -> [w590] mode=indexing
              tunnel: w587 -> [w588]
              tunnel: [w589] -> _
              n346 = call "MDI Close & deregister window.vi"("error in"=w588, "window"=w590) -> ("error out"=w589:errorcluster)  [unwired: 8 in]
            }
          }
          frame "Session:Close session" {
            n347 = Enqueue Element(queue=w592, element=Queue_steps_Main_applic."Session: close") -> ()  [unwired: 2 in, 3 out]
          }
          frame "Session:Save session as" {
            n348 = Enqueue Element(queue=w594, element=Queue_steps_Main_applic."Session: save as") -> ()  [unwired: 2 in, 3 out]
          }
          frame "Session:Save session" {
            n349 = Enqueue Element(queue=w596, element=Queue_steps_Main_applic."Session: save") -> ()  [unwired: 2 in, 3 out]
          }
          frame "Session:Load session:Browse" {
            n350 = flat-sequence {
              tunnel: [w600] -> w597
              tunnel: w598 -> [w600]
              frame #0 {
                n351 = local write "Session to load"(path "" ("Session to load")) -> ()
              }
            }
            n352 = Enqueue Element(queue=w597, element=Queue_steps_Main_applic."Session: load") -> ()  [unwired: 2 in, 3 out]
          }
          frame "File:Script" {
            n353 = Enqueue Element(queue=w603, element=Queue_steps_Main_applic."Script") -> ()  [unwired: 2 in, 3 out]
          }
          frame "File:TCP IP Script server" {
            n354 = Enqueue Element(queue=w605, element=Queue_steps_Main_applic."TCP IP script server") -> ()  [unwired: 2 in, 3 out]
          }
          frame "File:Import Register definition file" {
            n355 = Enqueue Element(queue=w607, element=Queue_steps_Main_applic."Import Excel table layout") -> ()  [unwired: 2 in, 3 out]
          }
          frame "Help:About..." {
            n356 = flat-sequence {
              tunnel: w609 -> [w614]
              tunnel: [w614] -> w608
              frame #0 {
                n357 = global read "RH PSTC MHCB2 CONSOLE global.vi" "RH PSTC MHCB2 CONSOLE main path"() -> (w611:path)
                n358 = Build Path(base path=w611, name or relative path="About\\PopUP_About.vi" ("append to path (empty)")) -> (appended path=w612:path)
                n359 = local write "Child to open"(w612) -> ()
              }
            }
            n360 = Enqueue Element(queue=w608, element=Queue_steps_Main_applic."MDI: open child") -> ()  [unwired: 2 in, 3 out]
          }
        }
      }
      event "Debugging info": Value Change {
        n361 = event-data() -> ()  [unwired: 1 in, 3 out]
        n362 = global write "MDI global.vi" "ContainerShowsDebugInfo"("Debugging info") -> ()
      }
    }
    n363 = local read "close"() -> (w478:bool)
  }
  n364 = case shown="True" "Do not use" {
    frame False {
    }
    frame True {
      n365 = call "MDI Overview.vi"() -> ()  [unwired: 1 in]
      n366 = call "Register definition UI.vi"() -> ()  [unwired: 12 in]
      n367 = call "Register graph UI.vi"() -> ()  [unwired: 1 in]
    }
  }
  n368 = call <vilib>:"Application Directory.vi"() -> ("Application Directory"=w11:path)
  n369 = property class="App"() -> ("App.Kind"=w13:T4)  [unwired: 2 in, 2 out]
  n370 = global write "RH PSTC MHCB2 CONSOLE global.vi" "RH PSTC MHCB2 CONSOLE main path"(w11) -> ()
  n371 = Not Equal?(x=T4."Development System" ("y"), y=w13) -> (x != y?=w15:bool)
  n372 = Build Path(base path=w11, name or relative path="Errors.log") -> (appended path=w9:path)
  n373 = Build Path(base path=w11, name or relative path="Error definitions.ini") -> (appended path=w12:path)
  n374 = Bundle By Name(cluster=T5 {"Window Lay-out"={"Title"="RH PSTC MHCB2 CONSOLE - error", "Show modal"=FALSE, "Default buttons"={"Ignore"=TRUE, "Retry"=FALSE, "Abort"=FALSE, "Abort application"=TRUE}}, "Logging"={"Enable"=TRUE, "Filepath"=path "", "Max # of lines in file"=1000}, "Error definition file"={"Filepath"=path ""}} ("Error notification settings"), "Logging.Filepath"=w9, "Error definition file.Filepath"=w12, "Window Lay-out.Show modal"=w15) -> (w7:T5)
  n375 = call "Error notification - engine.vi"("Error notification settings"=w7) -> ()
  n376 = call "Error notification - stop engine.vi"("error in (sync only)"=w3) -> ("error out"=w2:errorcluster)  [unwired: 10 in]
  n377 = property class="App"(error in=w2) -> ("App.Kind"=w4:T4)  [unwired: 1 in, 2 out]
  n378 = case shown="\"invalid app kind\", Default" w4 {
    selector: w4 -> [w616 w622]
    frame "invalid app kind", Default {
      n379 = flat-sequence {
        tunnel: w616 -> [w617]
        frame #0 {
          n380 = Format Into String(format string="App.Kind is %s'" ("message"), w617) -> (resulting string=w618:string)  [unwired: 2 in, 1 out]
          n381 = call "RH_WinDebugLogging.vi"("message"=w618, "prefix"="## RH PSTC MHCB2 CONSOLE ##") -> ()  [unwired: 6 in, 1 out]
        }
        frame #1 {
          n382 = Quit LabVIEW(quit? (T)=TRUE) -> ()
        }
      }
    }
    frame "Development System", "Evaluation" {
      n383 = Format Into String(format string="App.Kind is %s'" ("message"), w622) -> (resulting string=w623:string)  [unwired: 2 in, 1 out]
      n384 = call "RH_WinDebugLogging.vi"("message"=w623, "prefix"="## RH PSTC MHCB2 CONSOLE ##") -> ()  [unwired: 6 in, 1 out]
    }
  }
